vi "Get Paths Array GUI.vi"(9 "Types (string)":string[](array[string]), 10 "Data":string[](array[string])) -> ()   [LabVIEW 2013, in "Data.PGSQL.lvclass"]
uses:
  Data.PGSQL.lvclass
  Typedefs/Errors--enum.ctl
  <userlib>/_OpenG.lib/array/array.llb/Search 1D Array (String)__ogtk.vi
panel:
  out "selected_paths":string
  in  "UNDO LAST VALUE":bool
  out "Paths":string[](array[string])
  out "Message":string
  out "path_to_selected_column":string="llab_038:d001(TEST_TABLE--new_stuff(hippos))"
  out "selected_table":string="TEST_TABLE"
  in  "columns_list":i32(listbox)=1
  in  "tables_list":i32(listbox)=34
  in  "STOP":bool
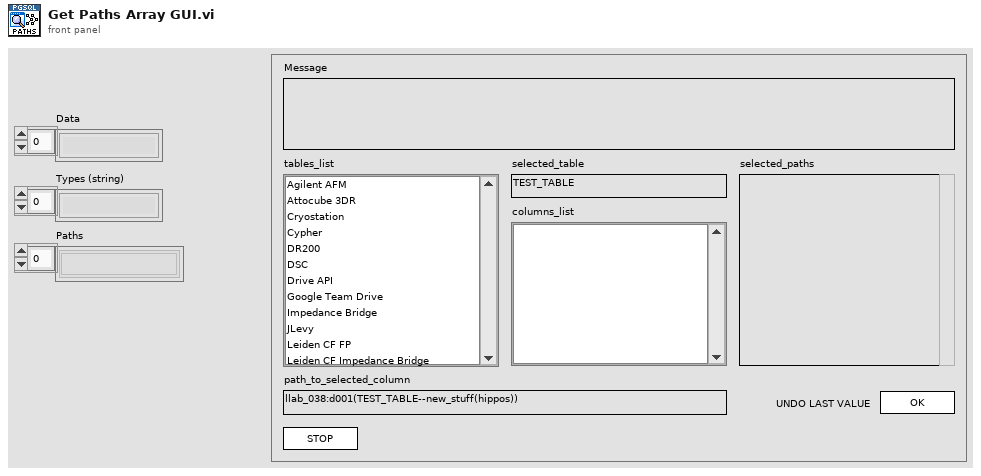
[diagram p1: front panel]
types:
  T1 = enum32{"Invalid", "Standard", "Closed", "Hidden", "Minimized", "Maximized"}
  T2 = enum32{"invalid app kind", "Development System", "Run Time System", "Student Edition", "Embedded LabVIEW", "Evaluation", "Custom"}
  T3 = typedef "Data.PGSQL.lvclass/Errors--enum.ctl" = enum16{"0: None", "5005: Path Type Not Supported", "5006: Number of Variables", "5008: Cannot write two data points", "5030: Start and End Times Identical", "5031: Input is not wholly", "5033: Bad path or paths", "5040: Invalid Instrument Name", "5050: Column can only hold string", "5051 Column can only hold bool", "5052: Column can only hold double", "5053: Column can only hold int"}
  T4 = cluster{"Core":cluster{"Current VI Reference":refnum<vi>, "Close Panel on Exit?":bool}, "Data.PG in":refnum<class "Data.PGSQL.lvclass">, "table names":string[], "table paths":string[], "column names":string[], "column units":string[], "column paths":string[], "new table name":string, "new column name":string, "new column data type":string, "new column units":string, "selected table":string, "selected column":string, "selected table path":string, "selected column path":string, "selected column units":string, "Paths array":string[], "Current Index":i32, "Data":string[], "Types (string)":string[]}
  T5 = cluster{"Current VI Reference":refnum<vi>, "Close Panel on Exit?":bool}
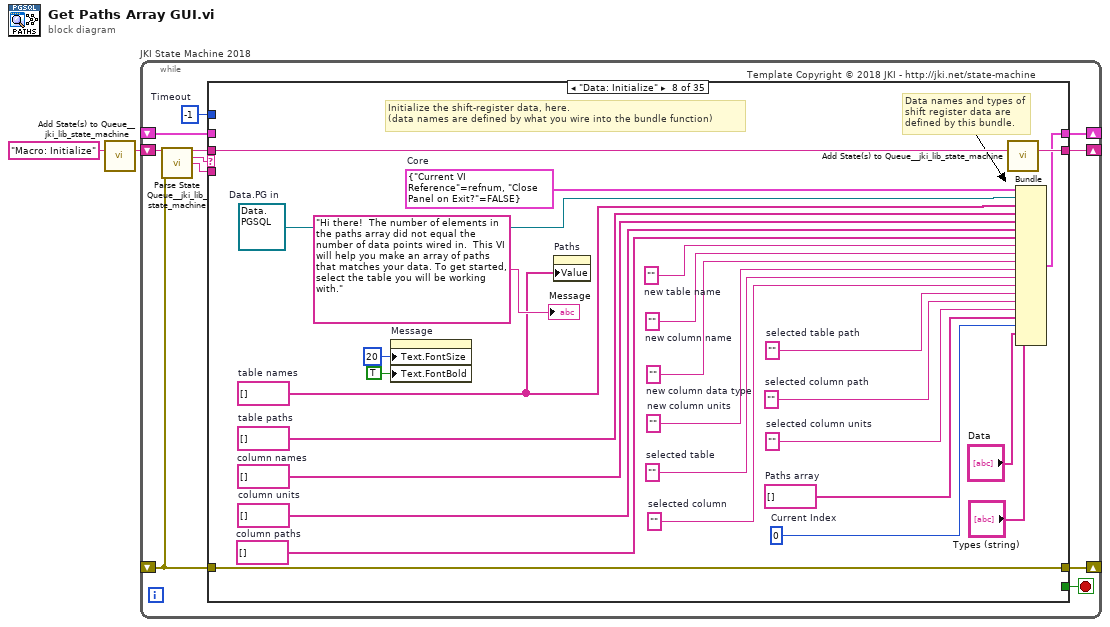
[diagram p0: block diagram]
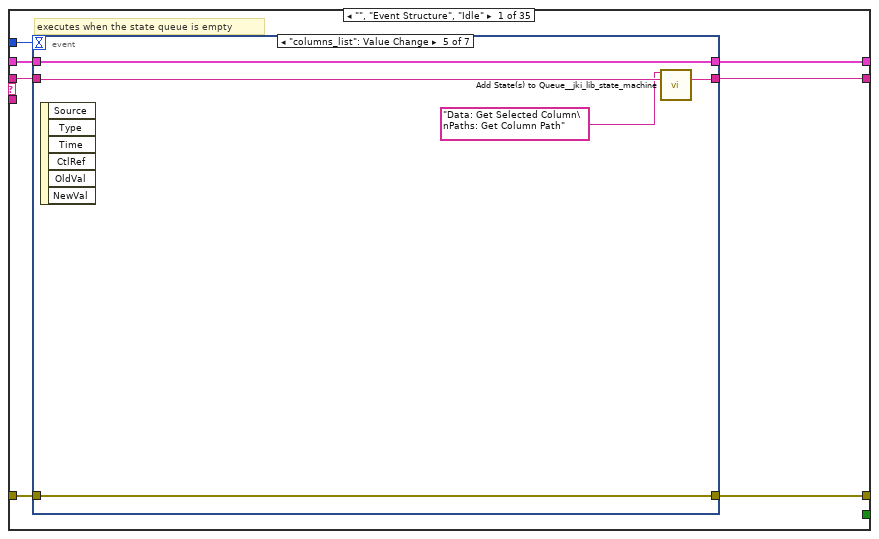
[diagram p2: hidden frame]
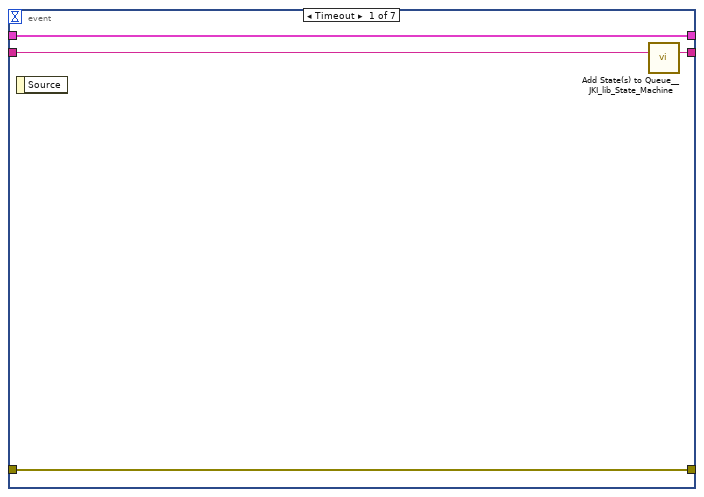
[diagram p3: hidden frame]
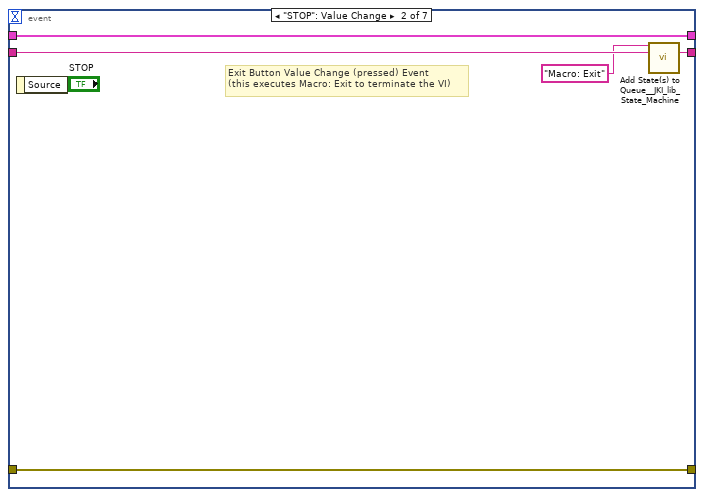
[diagram p4: hidden frame]
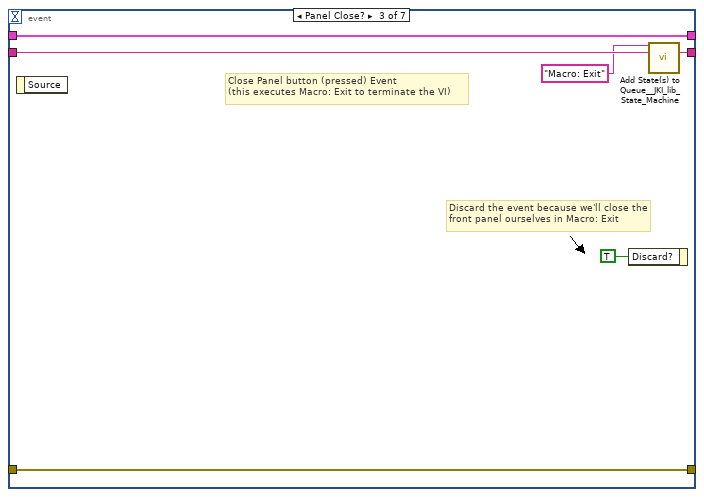
[diagram p5: hidden frame]
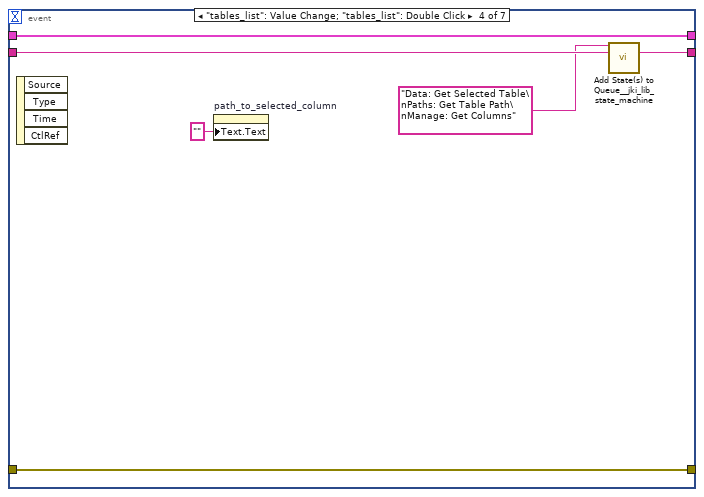
[diagram p6: hidden frame]
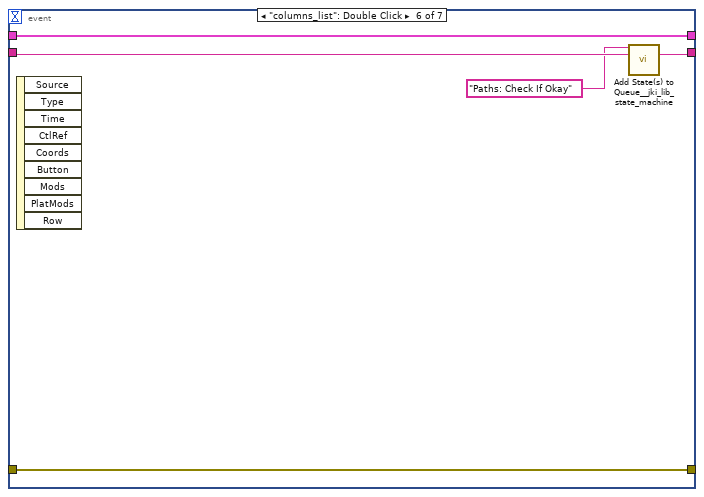
[diagram p7: hidden frame]
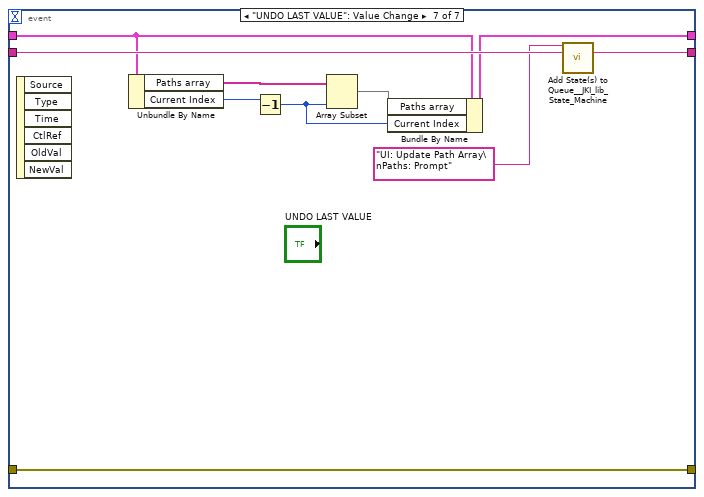
[diagram p8: hidden frame]
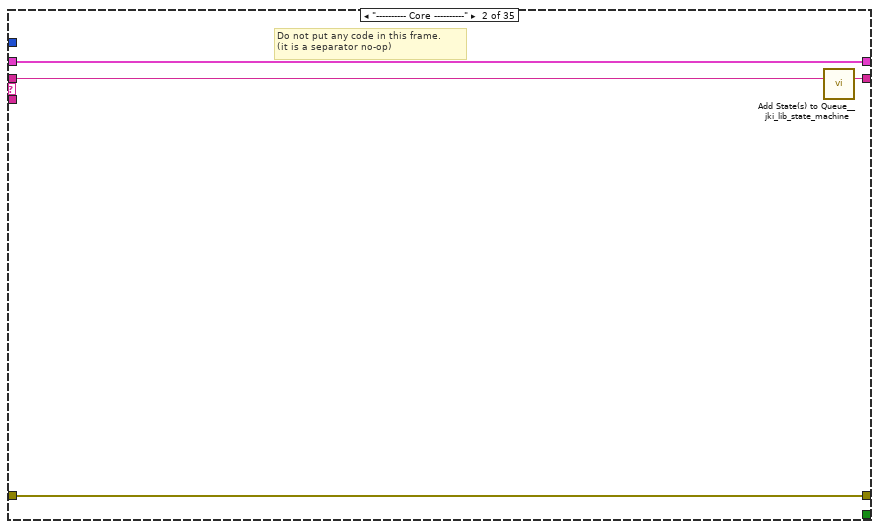
[diagram p9: hidden frame]
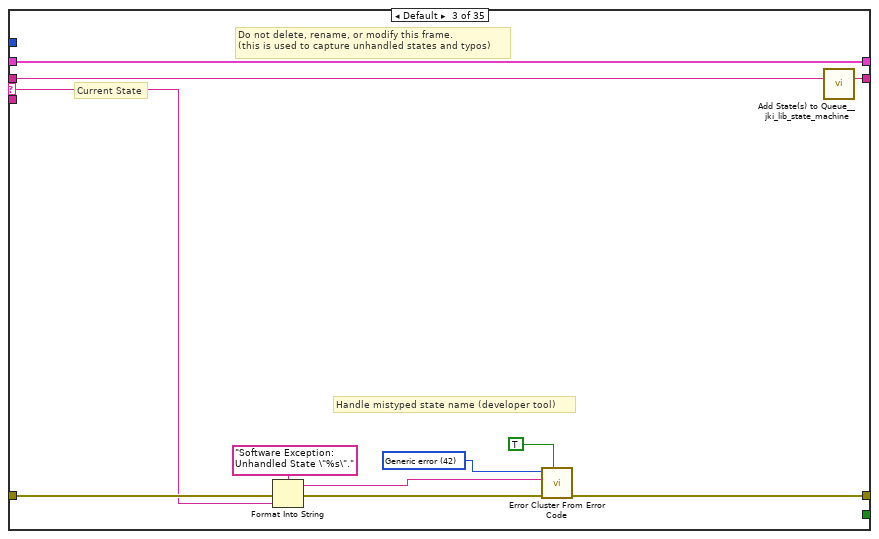
[diagram p10: hidden frame]
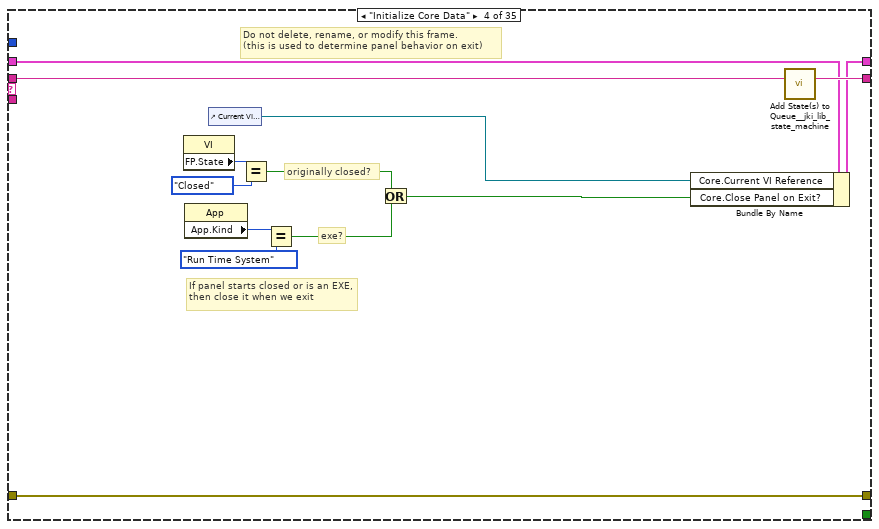
[diagram p11: hidden frame]
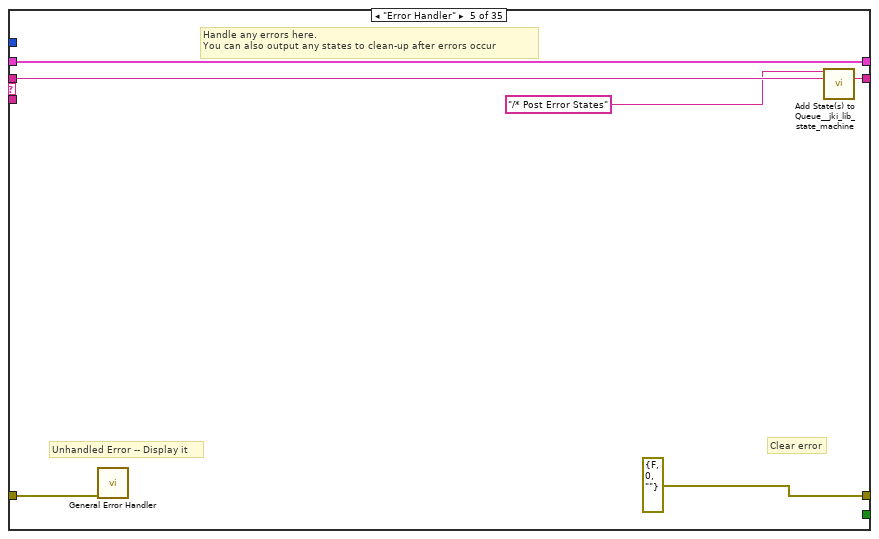
[diagram p12: hidden frame]
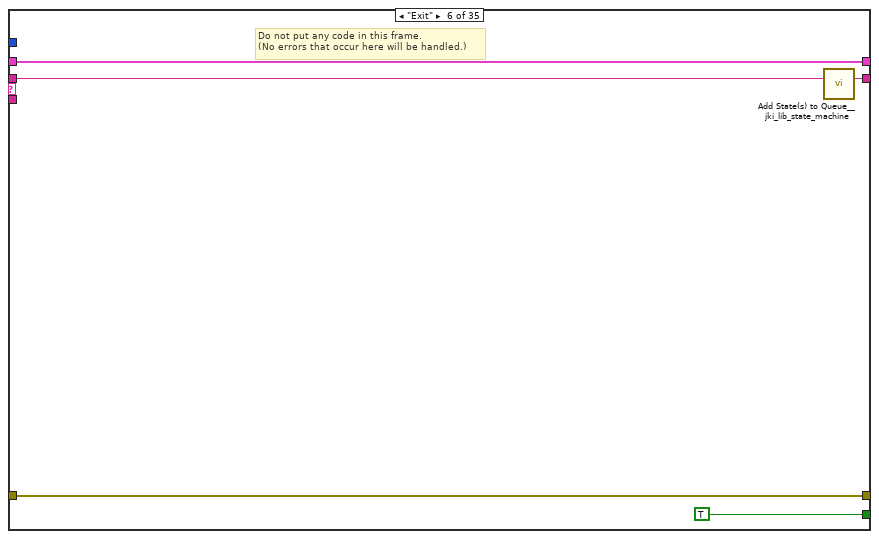
[diagram p13: hidden frame]
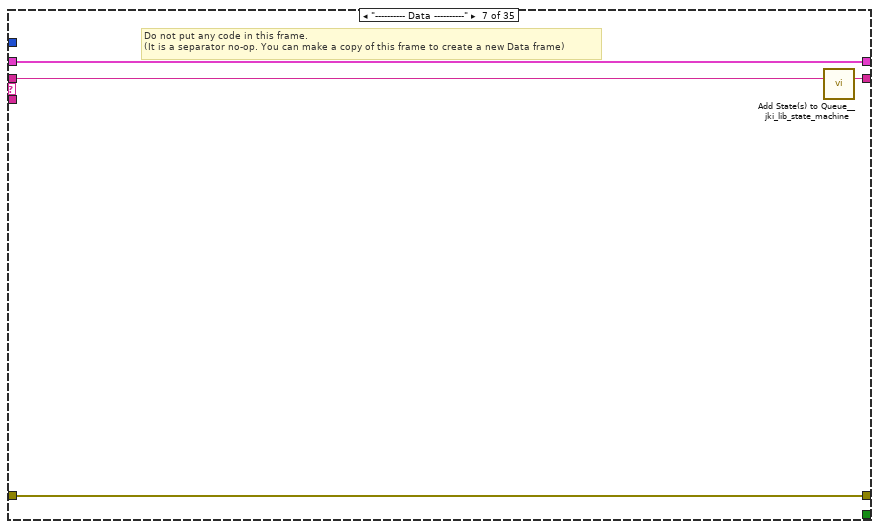
[diagram p14: hidden frame]
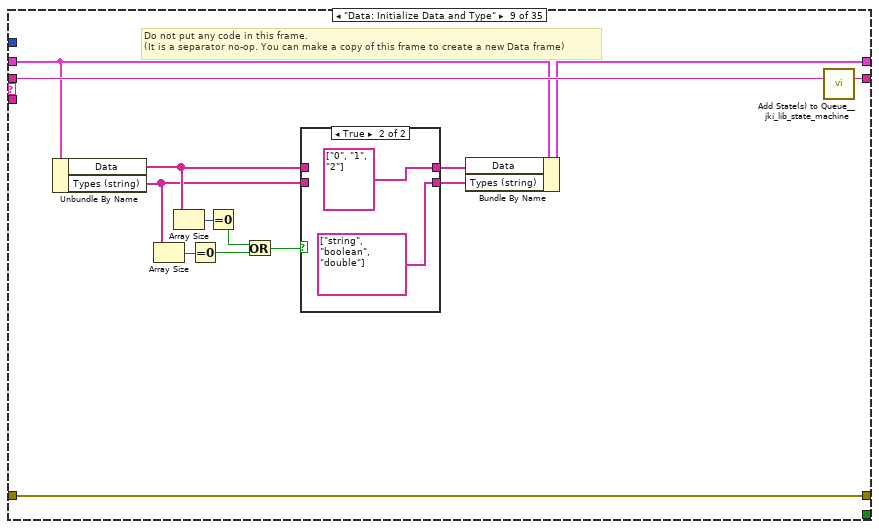
[diagram p15: hidden frame]
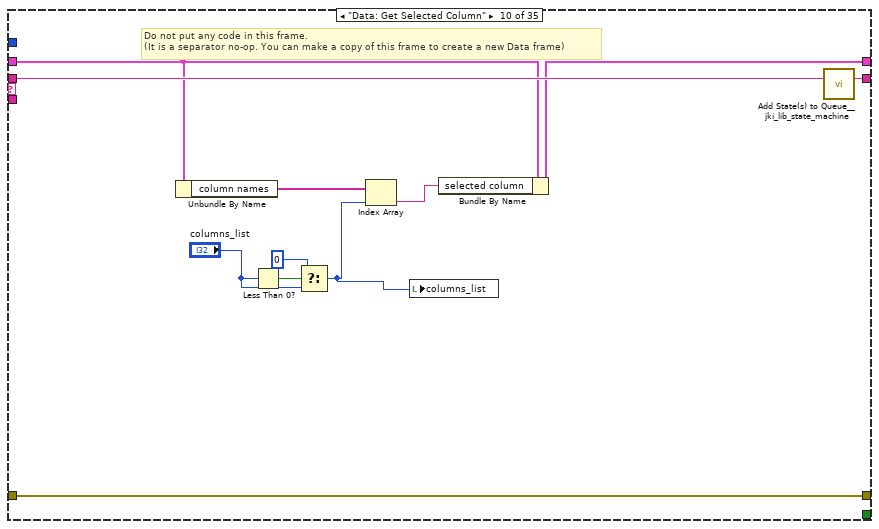
[diagram p17: hidden frame]
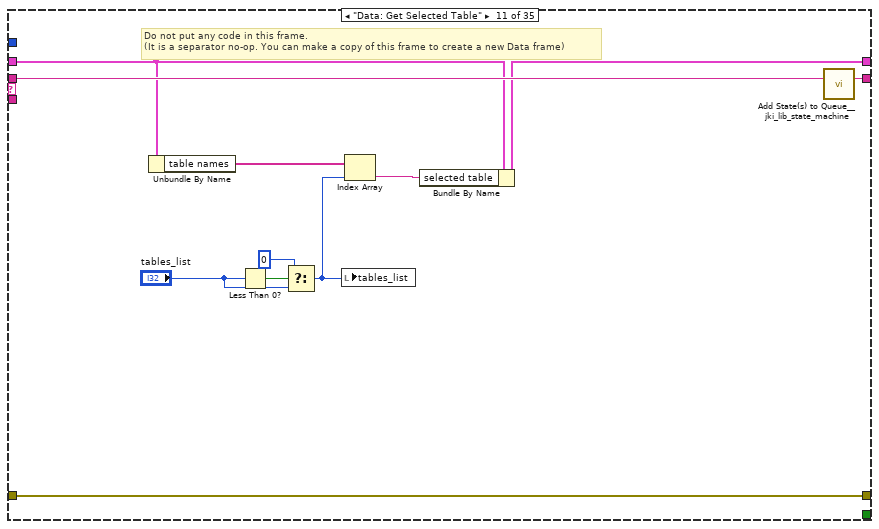
[diagram p18: hidden frame]
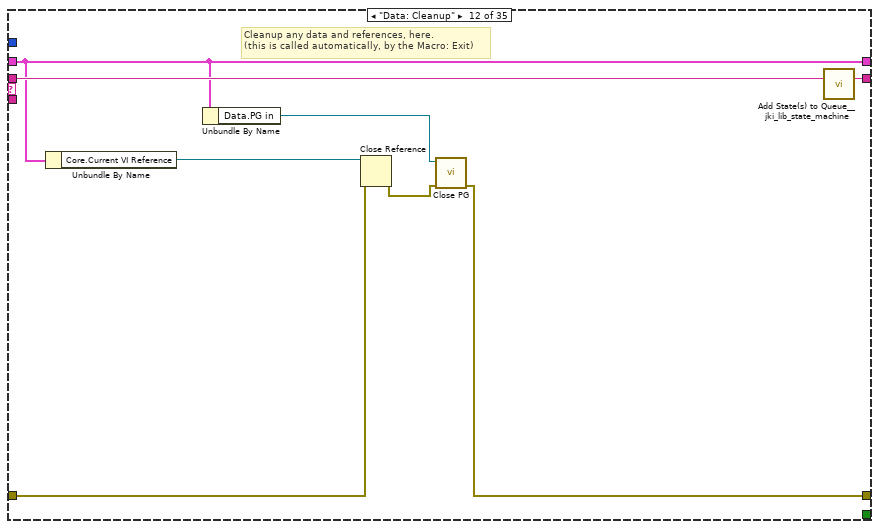
[diagram p19: hidden frame]
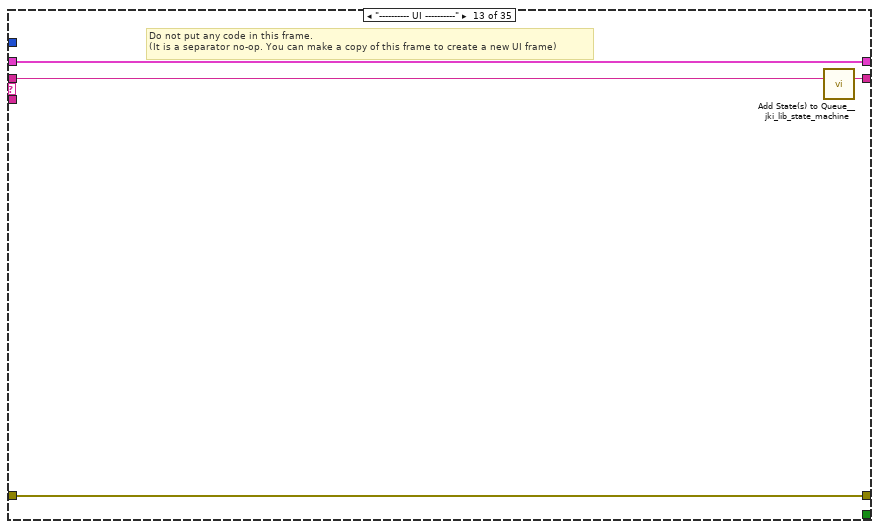
[diagram p20: hidden frame]
diagram:
  n1 = call <vilib>:"Add State(s) to Queue__jki_lib_state_machine.vi"("State(s) in (\"\")"="Macro: Initialize") -> ("States Out"=w2:string)  [unwired: 14 in]
  n2 = while "JKI State Machine 2018" {
    shift-right: [w6] -> _
    shift-left: _ -> [w5]
    shift-right: [w9] -> _
    shift-left: _ -> [w3]
    shift-right: [w8] -> _
    shift-left: w2 -> [w10]
    stop <- w7 stop-if-true
    w4 = -1  # Timeout
    # "Template Copyright © 2018 JKI - http://jki.net/state-machine"
    n3 = call <vilib>:"Parse State Queue__jki_lib_state_machine.vi"("State Queue"=w10, "Error In (no error)"=w3) -> ("Remaining States"=w12:string, "Current State"=w13:string, "Arguments"=w11:string)  [unwired: 11 in]
    n4 = case shown="\"Data: Initialize\"" w13 {
      selector: w13 -> [_ _ w66 _ _ _ _ _ _ _ _ _ _ _ _ _ _ _ _ _ _ _ _ _ _ _ _ _ _ _ _ _ _ _ _]
      tunnel: w12 -> [w20 w65 w70 w89 w95 w100 w104 w131 w145 w160 w171 w179 w183 w194 w202 w208 w219 w291 w296 w305 w309 w314 w324 w328 w337 w350 w354 w360 w368 w372 w381 w395 w406 w425 w461]
      tunnel: w11 -> [_ _ _ _ _ _ _ _ _ _ _ _ _ _ _ w203 w213 _ _ _ _ _ _ _ _ _ _ _ _ _ _ _ _ _ _]
      tunnel: w5 -> [w18 w62 w68 w82 w92 w98 w101 _ w142 w155 w166 w173 w180 w186 w197 w206 w215 w288 w293 w302 w306 w311 w321 w325 w335 w348 w351 w358 w366 w369 w379 w393 w403 w419 w459]
      tunnel: [w17 w63 w72 w86 errorcluster {"status"=FALSE, "code"=0, "source"=""} ("error out") w97 w102 w128 w143 w158 w169 w174 w181 w185 w200 w204 w216 w289 w294 w303 w307 w312 w322 w326 w331 w344 w352 w355 w362 w370 w375 w383 w404 w423 w443] -> w9
      tunnel: w3 -> [w16 w63 w71 w86 w91 w97 w102 w128 w143 w158 w169 w176 w181 w192 w200 w205 w217 w289 w294 w303 w307 w312 w322 w326 w332 w345 w352 w356 w361 w370 w376 w384 w404 w423 w440]
      tunnel: [w19 w64 w69 w88 w94 w99 w103 w130 w144 w159 w170 w178 w182 w193 w201 w207 w218 w290 w295 w304 w308 w313 w323 w327 w336 w349 w353 w359 w367 w371 w380 w394 w405 w424 w460] -> w8
      tunnel: [_ _ _ _ _ TRUE _ _ _ _ _ _ _ _ _ _ _ _ _ _ _ _ _ _ _ _ _ _ _ _ _ _ _ _ _] -> w7
      tunnel: [w15 w62 w68 w87 w92 w98 w101 w129 w141 w156 w165 w173 w180 w186 w197 w206 w215 w288 w293 w302 w306 w311 w321 w325 w334 w347 w351 w358 w365 w369 w373 w385 w403 w408 w459] -> w6
      tunnel: w4 -> [w14 _ _ _ _ _ _ _ _ _ _ _ _ _ _ _ _ _ _ _ _ _ _ _ _ _ _ _ _ _ _ _ _ _ _]
      frame "", "Event Structure", "Idle" {
        # "executes when the state queue is empty"
        n5 = event shown="[4] \"columns_list\": Value Change" {
          selector: _ -> [_ _ _ _ _ _ _]
          dyn-events: _ -> [_ _ _ _ _ _ _]
          timeout: w14 -> [_ _ _ _ _ _ _]
          tunnel: w20 -> [w24 w29 w35 w39 w44 w49 w59]
          tunnel: [w23 w28 w34 w40 w45 w50 w60] -> w19
          tunnel: w18 -> [w21 w26 w32 w36 w46 w48 w56]
          tunnel: [w22 w27 w33 w41 w42 w51 w61] -> w17
          tunnel: w16 -> [w22 w27 w33 w41 w42 w51 w61]
          tunnel: [w21 w26 w32 w36 w46 w48 w55] -> w15
          event Timeout {
            n6 = event-data() -> ()  [unwired: 1 in, 1 out]
            n7 = call <vilib>:"Add State(s) to Queue__JKI_lib_State_Machine.vi"("State(s) in (\"\")"=w24) -> ("States Out"=w23:string)  [unwired: 14 in]
          }
          event "STOP": Value Change {
            # "Exit Button Value Change (pressed) Event\n(this executes Macro: Exit to terminate the VI)"
            n8 = event-data() -> ()  [unwired: 1 in, 1 out]
            n9 = call <vilib>:"Add State(s) to Queue__JKI_lib_State_Machine.vi"("State(s) in Front (\"\")"="Macro: Exit", "State(s) in (\"\")"=w29) -> ("States Out"=w28:string)  [unwired: 13 in]
          }
          event Panel Close? {
            # "Discard the event because we'll close the front panel ourselves in Macro: Exit"
            # "Close Panel button (pressed) Event\n(this executes Macro: Exit to terminate the VI)"
            n10 = event-data() -> ()  [unwired: 1 in, 1 out]
            n11 = event-data("Discard?"=TRUE) -> ()  [unwired: 1 in, 1 out]
            n12 = call <vilib>:"Add State(s) to Queue__JKI_lib_State_Machine.vi"("State(s) in Front (\"\")"="Macro: Exit", "State(s) in (\"\")"=w35) -> ("States Out"=w34:string)  [unwired: 13 in]
          }
          event "tables_list": Value Change; "tables_list": Double Click {
            n13 = event-data() -> ()  [unwired: 1 in, 4 out]
            n14 = property on="path_to_selected_column" class="Str"("Text.Text"="") -> ()  [unwired: 2 in, 2 out]
            n15 = call <vilib>:"Add State(s) to Queue__jki_lib_state_machine.vi"("State(s) in Front (\"\")"="Data: Get Selected Table\nPaths: Get Table Path\nManage: Get Columns" ("State(s) in Front (\"\")"), "State(s) in (\"\")"=w39) -> ("States Out"=w40:string)  [unwired: 13 in]
          }
          event "columns_list": Value Change {
            n16 = event-data() -> ()  [unwired: 1 in, 6 out]
            n17 = call <vilib>:"Add State(s) to Queue__jki_lib_state_machine.vi"("State(s) in Front (\"\")"="Data: Get Selected Column\nPaths: Get Column Path", "State(s) in (\"\")"=w44) -> ("States Out"=w45:string)  [unwired: 13 in]
          }
          event "columns_list": Double Click {
            n18 = event-data() -> ()  [unwired: 1 in, 9 out]
            n19 = call <vilib>:"Add State(s) to Queue__jki_lib_state_machine.vi"("State(s) in Front (\"\")"="Paths: Check If Okay" ("State(s) in Front (\"\")"), "State(s) in (\"\")"=w49) -> ("States Out"=w50:string)  [unwired: 13 in]
          }
          event "UNDO LAST VALUE": Value Change {
            n20 = event-data() -> ()  [unwired: 1 in, 6 out]
            n21 = Unbundle By Name(w56) -> ("Paths array"=w57:string[], "Current Index"=w58:i32)
            n22 = Decrement(x=w58) -> (x-1=w54:i32)
            n23 = Array Subset(array=w57, length=w54) -> (w53:string[])  [unwired: 1 in]
            n24 = Bundle By Name(cluster=w56, "Paths array"=w53, "Current Index"=w54) -> (w55:T4)
            n25 = call <vilib>:"Add State(s) to Queue__JKI_lib_State_Machine.vi"("State(s) in Front (\"\")"="UI: Update Path Array\nPaths: Prompt" ("State(s) in Front (\"\")"), "State(s) in (\"\")"=w59) -> ("States Out"=w60:string)  [unwired: 13 in]
          }
        }
      }
      frame "---------- Core ----------" {
        # "Do not put any code in this frame.\n(it is a separator no-op)"
        n26 = call <vilib>:"Add State(s) to Queue__jki_lib_state_machine.vi"("State(s) in (\"\")"=w65) -> ("States Out"=w64:string)  [unwired: 14 in]
      }
      frame Default {
        w75 = 42 items=["No error", "Argument error", "Memory is full", "Out of zone", "End of file", "File already open", "Generic file I/O error", "File not found", "File permission error", "Disk is full", "Duplicate path", "Too many files open", "System feature not enabled", "Resource file not found", "Cannot add resource", "Resource not found", "Image not found", "Image memory error", "Pen does not exist", "Config type invalid", "Config token not found", "Config parse error", "Config memory error", "Bad external code format", "Bad external code offset", "External code not present", "Null window", "Destroy window error", "Null menu", "Print aborted", "Bad print record", "Print driver error", "Windows error during printing", "Memory error during printing", "Print dialog error", "Generic print error", "Invalid device refnum", "Device not found", "Device parameter error", "Device unit error", "Cannot open device", "Device call aborted", "Generic error", "Cancelled by user", "Object ID too low", "Object ID too high", "Object not in heap", "Unknown heap", "Unknown object (invalid DefProc)", "Unknown object (DefProc not in table)", "Message out of range", "Invalid (null) method", "Unknown message", "Manager call not supported", "Bad address", "Network operation in progress", "Network operation timed out", "Connection is busy", "Network attribute not supported", "Network error", "Address in use", "System out of memory", "Connection aborted", "Connection refused", "Not connected", "Already connected", "Connection closed", "Initialization error (interapplication manager)", "Bad occurrence", "Wait on unbound occurrence handler", "Occurrence queue overflow", "Datalog type conflict", "Unused", "Unrecognized type (interapplication manager)", "Memory corrupt", "Failed to make temporary DLL", "Old CIN version", "Drag socket not found", "Failed to load drop-object", "Failed to register OLE object", "Failed to release OLE object", "Format specifier type mismatch", "Unknown format specifier", "Too few format specifiers", "Too many format specifiers", "Scan failed", "Newer CIN version", "Error converting to variant", "Runtime menu error", "Password tampered", "Variant attribute not found", "Incompatible variant data type", "Event data is not available", "Event Store is not present", "Occurrence is not found", "Event Queue is not created", "Event info is not available", "Refnum passed is NULL", "Error retrieving Class GUID", "Error retrieving CoClass GUID", "Error retrieving TypeLib GUID.", "Bad built application magic bytes.", "Specific driver is different from the specific driver associated with the Logical Name.", "There is no session opened to the class driver.", "Max Error", "MAX - Error with config objects", "MAX - Error loading configuration", "MAX - Group not supported"]
        # "Current State"
        # "Do not delete, rename, or modify this frame.\n(this is used to capture unhandled states and typos)"
        # "Handle mistyped state name (developer tool)"
        n27 = Format Into String(format string="Software Exception: Unhandled State \"%s\"." ("message"), error in=w71, w66) -> (resulting string=w74:string, error out=w73:errorcluster)  [unwired: 1 in]
        n28 = call <vilib>:"Error Cluster From Error Code.vi"("show call chain? (False)"=TRUE, "error in (no error)"=w73, "error message (\"\")"=w74, "error code (0)"=w75) -> ("error out"=w72:errorcluster)  [unwired: 5 in]
        n29 = call <vilib>:"Add State(s) to Queue__jki_lib_state_machine.vi"("State(s) in (\"\")"=w70) -> ("States Out"=w69:string)  [unwired: 14 in]
      }
      frame "Initialize Core Data" {
        # "Do not delete, rename, or modify this frame.\n(this is used to determine panel behavior on exit)"
        # "originally closed?"
        # "exe?"
        # "If panel starts closed or is an EXE, then close it when we exit"
        n30 = property class="VI"() -> ("FP.State"=w79:T1)  [unwired: 2 in, 2 out]
        n31 = property class="App"() -> ("App.Kind"=w85:T2)  [unwired: 2 in, 2 out]
        n32 = control-ref of="Current VI Reference"() -> (w80:refnum<vi>)
        n33 = Equal?(x=w79, y=T1."Closed" ("Front Panel Window:State")) -> (x = y?=w77:bool)
        n34 = Equal?(x=w85, y=T2."Run Time System" ("Application:Kind")) -> (x = y?=w83:bool)
        n35 = Or(x=w77, y=w83) -> (x .or. y?=w81:bool)
        n36 = Bundle By Name(cluster=w82, "Core.Current VI Reference"=w80, "Core.Close Panel on Exit?"=w81) -> (w87:T4)
        n37 = call <vilib>:"Add State(s) to Queue__jki_lib_state_machine.vi"("State(s) in (\"\")"=w89) -> ("States Out"=w88:string)  [unwired: 14 in]
      }
      frame "Error Handler" {
        # "Unhandled Error -- Display it"
        # "Handle any errors here.\nYou can also output any states to clean-up after errors occur"
        # "Clear error"
        n38 = call <vilib>:"General Error Handler.vi"("error in (no error)"=w91) -> ()  [unwired: 10 in, 5 out]
        n39 = call <vilib>:"Add State(s) to Queue__jki_lib_state_machine.vi"("State(s) in Front (\"\")"="/* Post Error States", "State(s) in (\"\")"=w95) -> ("States Out"=w94:string)  [unwired: 13 in]
      }
      frame "Exit" {
        # "Do not put any code in this frame.\n(No errors that occur here will be handled.)"
        n40 = call <vilib>:"Add State(s) to Queue__jki_lib_state_machine.vi"("State(s) in (\"\")"=w100) -> ("States Out"=w99:string)  [unwired: 14 in]
      }
      frame "---------- Data ----------" {
        # "Do not put any code in this frame.\n(It is a separator no-op. You can make a copy of this frame to create a new Data frame)"
        n41 = call <vilib>:"Add State(s) to Queue__jki_lib_state_machine.vi"("State(s) in (\"\")"=w104) -> ("States Out"=w103:string)  [unwired: 14 in]
      }
      frame "Data: Initialize" {
        w112 = 0  # Current Index
        w113 = string[] []  # Paths array
        w114 = ""  # selected column units
        w105 = ""  # selected column path
        w115 = ""  # selected table path
        w116 = ""  # selected column
        w117 = ""  # selected table
        w118 = ""  # new column units
        w119 = ""  # new column data type
        w120 = ""  # new column name
        w121 = ""  # new table name
        w122 = string[] []  # column paths
        w123 = string[] []  # column units
        w124 = string[] []  # column names
        w125 = string[] []  # table paths
        w106 = string[] []  # table names
        w126 = refnum<class "Data.PGSQL.lvclass"> refnum  # Data.PG in
        w127 = T5 {"Current VI Reference"=refnum, "Close Panel on Exit?"=FALSE}  # Core
        # "Data names and types of shift register data are defined by this bundle."
        # "Initialize the shift-register data, here.\n(data names are defined by what you wire into the bundle function)"
        n42 = property on="Message" class="Str"("Text.FontSize"=u32 20 ("Text.Font:Size"), "Text.FontBold"=TRUE ("Text.Font:Bold")) -> ()  [unwired: 2 in, 2 out]
        n43 = property on="Paths" class="Arr (strict)"("Value"=w106) -> ()  [unwired: 2 in, 2 out]
        n44 = call <vilib>:"Add State(s) to Queue__jki_lib_state_machine.vi"("State(s) in (\"\")"=w131) -> ("States Out"=w130:string)  [unwired: 14 in]
        n45 = Bundle("Core"=w127, "Data.PG in"=w126, "table names"=w106, "table paths"=w125, "column names"=w124, "column units"=w123, "column paths"=w122, "new table name"=w121, "new column name"=w120, "new column data type"=w119, "new column units"=w118, "selected table"=w117, "selected column"=w116, "selected table path"=w115, "selected column path"=w105, "selected column units"=w114, "Paths array"=w113, "Current Index"=w112, "Data"="Data", "Types (string)"="Types (string)") -> (w129:T4)  [unwired: 1 in]
        "Message" <- "Hi there!  The number of elements in the paths array did not equal the number of data points wired in.  This VI will help you make an array of paths that matches your data. To get started, select the table you will be working with." ("String")
      }
      frame "Data: Initialize Data and Type" {
        # "Do not put any code in this frame.\n(It is a separator no-op. You can make a copy of this frame to create a new Data frame)"
        n46 = Unbundle By Name(w142) -> ("Data"=w134:string[], "Types (string)"=w132:string[])
        n47 = Array Size(array=w132) -> (size(s)=w139:i32)
        n48 = Array Size(array=w134) -> (size(s)=w140:i32)
        n49 = Equal To 0?(x=w139) -> (x = 0?=w137:bool)
        n50 = Equal To 0?(x=w140) -> (x = 0?=w138:bool)
        n51 = Or(x=w138, y=w137) -> (x .or. y?=w136:bool)
        n52 = case shown="True" w136 {
          tunnel: [w147 string[] ["0", "1", "2"] ("Data")] -> w135
          tunnel: w134 -> [w147 _]
          tunnel: [w146 string[] ["string", "boolean", "double"] ("Types (string)")] -> w133
          tunnel: w132 -> [w146 _]
          frame False {
          }
          frame True {
          }
        }
        n53 = Bundle By Name(cluster=w142, "Data"=w135, "Types (string)"=w133) -> (w141:T4)
        n54 = call <vilib>:"Add State(s) to Queue__jki_lib_state_machine.vi"("State(s) in (\"\")"=w145) -> ("States Out"=w144:string)  [unwired: 14 in]
      }
      frame "Data: Get Selected Column" {
        # "Do not put any code in this frame.\n(It is a separator no-op. You can make a copy of this frame to create a new Data frame)"
        n55 = Unbundle By Name(w155) -> ("column names"=w157:string[])
        n56 = Less Than 0?(x="columns_list") -> (x < 0?=w153:bool)
        n57 = Select(t=0, s=w153, f="columns_list") -> (s? t:f=w150:i32)
        n58 = Index Array(array=w157, index=w150) -> (element=w151:string)
        n59 = local write "columns_list"(w150) -> ()
        n60 = Bundle By Name(cluster=w155, "selected column"=w151) -> (w156:T4)
        n61 = call <vilib>:"Add State(s) to Queue__jki_lib_state_machine.vi"("State(s) in (\"\")"=w160) -> ("States Out"=w159:string)  [unwired: 14 in]
      }
      frame "Data: Get Selected Table" {
        # "Do not put any code in this frame.\n(It is a separator no-op. You can make a copy of this frame to create a new Data frame)"
        n62 = Unbundle By Name(w166) -> ("table names"=w167:string[])
        n63 = Less Than 0?(x="tables_list") -> (x < 0?=w163:bool)
        n64 = Select(t=0, s=w163, f="tables_list") -> (s? t:f=w161:i32)
        n65 = local write "tables_list"(w161) -> ()
        n66 = Index Array(array=w167, index=w161) -> (element=w168:string)
        n67 = Bundle By Name(cluster=w166, "selected table"=w168) -> (w165:T4)
        n68 = call <vilib>:"Add State(s) to Queue__jki_lib_state_machine.vi"("State(s) in (\"\")"=w171) -> ("States Out"=w170:string)  [unwired: 14 in]
      }
      frame "Data: Cleanup" {
        # "Cleanup any data and references, here.\n(this is called automatically, by the Macro: Exit)"
        n69 = Unbundle By Name(w173) -> ("Core.Current VI Reference"=w177:refnum<vi>)
        n70 = Unbundle By Name(w173) -> ("Data.PG in"=w172:refnum<class "Data.PGSQL.lvclass">)
        n71 = Close Reference(reference=w177, error in (no error)=w176) -> (error out=w175:errorcluster)
        n72 = call-dynamic "Close PG.vi"("error in (no error)"=w175, "Data.PG in"=w172) -> ("error out"=w174:errorcluster)  [unwired: 8 in, 1 out]
        n73 = call <vilib>:"Add State(s) to Queue__jki_lib_state_machine.vi"("State(s) in (\"\")"=w179) -> ("States Out"=w178:string)  [unwired: 14 in]
      }
      frame "---------- UI ----------" {
        # "Do not put any code in this frame.\n(It is a separator no-op. You can make a copy of this frame to create a new UI frame)"
        n74 = call <vilib>:"Add State(s) to Queue__jki_lib_state_machine.vi"("State(s) in (\"\")"=w183) -> ("States Out"=w182:string)  [unwired: 14 in]
      }
      frame "UI: Initialize" {
        w184 = "" ("Text.Text")
        # "Initialize the User Interface, here.\n(this is called automatically, by the Macro: Init)"
        n75 = Unbundle By Name(w186) -> ("table names"=w191:string[], "column names"=w190:string[], "selected table"=→"selected_table":string)
        n76 = call <userlib>:"Fit VI window to Largest Dec__ogtk.vi"("error in (no error)"=w192) -> ("error out"=w185:errorcluster)  [unwired: 5 in, 1 out]
        n77 = property on="tables_list" class="LstBox (strict)"("Item Names"=w191) -> ()  [unwired: 2 in, 2 out]
        n78 = Build Array(0) -> (w187:i32[])
        n79 = property on="path_to_selected_column" class="Str"("Text.Text"=w184) -> ()  [unwired: 2 in, 2 out]
        n80 = local write "selected_paths"(w184) -> ()
        n81 = property on="Paths" class="Arr (strict)"("Index Values"=w187) -> ()  [unwired: 2 in, 2 out]
        n82 = property on="columns_list" class="LstBox (strict)"("Item Names"=w190) -> ()  [unwired: 2 in, 2 out]
        n83 = call <vilib>:"Add State(s) to Queue__jki_lib_state_machine.vi"("State(s) in (\"\")"=w194) -> ("States Out"=w193:string)  [unwired: 14 in]
      }
      frame "UI: Update" {
        # "Initialize the User Interface, here.\n(this is called automatically, by the Macro: Init)"
        n84 = Unbundle By Name(w197) -> ("table names"=w199:string[], "column names"=w198:string[], "selected table"=w195:string, "selected column"=w196:string)
        n85 = local write "selected_table"(w195) -> ()
        n86 = property on="tables_list" class="LstBox (strict)"("Item Names"=w199) -> ()  [unwired: 2 in, 2 out]
        n87 = property on="path_to_selected_column" class="Str"("Text.Text"=w196) -> ()  [unwired: 2 in, 2 out]
        n88 = property on="columns_list" class="LstBox (strict)"("Item Names"=w198) -> ()  [unwired: 2 in, 2 out]
        n89 = call <vilib>:"Add State(s) to Queue__jki_lib_state_machine.vi"("State(s) in (\"\")"=w202) -> ("States Out"=w201:string)  [unwired: 14 in]
      }
      frame "UI: Cursor Set" {
        # "Argument"
        # "Set and Unset Cursor Busy.\n(Usage: \"UI: Cursor Set >> Busy|Idle\")"
        n90 = case shown="\"Idle\", Default" w203 {
          tunnel: w205 -> [w210 w212]
          tunnel: [w209 w211] -> w204
          frame "Idle", Default {
            n91 = call <vilib>:"Unset Busy.vi"("error in (no error)"=w210) -> ("error out"=w209:errorcluster)  [unwired: 10 in]
          }
          frame "Busy" {
            n92 = call <vilib>:"Set Busy.vi"("error in (no error)"=w212) -> ("error out"=w211:errorcluster)  [unwired: 9 in, 1 out]
          }
        }
        n93 = call <vilib>:"Add State(s) to Queue__jki_lib_state_machine.vi"("State(s) in (\"\")"=w208) -> ("States Out"=w207:string)  [unwired: 14 in]
      }
      frame "UI: Front Panel State" {
        # "Argument"
        # "Set Front Panel Open or Closed\n(Usage: \"UI: Front Panel State >> Open|Close\")"
        n94 = Unbundle By Name(w215) -> ("Core.Current VI Reference"=w214:refnum<vi>)
        n95 = case shown="\"Maximize\", \"Maximized\"" w213 {
          tunnel: w217 -> [w225 w240 w251 w264 w277]
          tunnel: [w227 w241 w253 w266 w279] -> w216
          tunnel: w214 -> [w226 w238 w252 w265 w278]
          frame "Open", "Standard", Default {
            w220 = T1."Standard" ("State")
            n96 = property class="VI"(reference=w226, error in=w225) -> (reference out=w223:refnum<vi>, error out=w224:errorcluster, "FP.State"=w222:T1)
            n97 = Not Equal?(x=w222, y=w220) -> (x != y?=w221:bool)
            n98 = case shown="True" w221 {
              tunnel: [w231 w233] -> w227
              tunnel: w224 -> [w230 w233]
              tunnel: w223 -> [w229 _]
              tunnel: w220 -> [w228 _]
              frame True {
                n99 = invoke class="VI" method="FP.Open"(reference=w229, error in=w230, "Activate"=TRUE, "State"=w228) -> (error out=w231:errorcluster)  [unwired: 1 in, 4 out]
              }
              frame False {
              }
            }
          }
          frame "Close", "Closed" {
            n100 = property class="VI"(reference=w238, error in=w240) -> (reference out=w237:refnum<vi>, error out=w239:errorcluster, "FP.State"=w235:T1)
            n101 = Not Equal?(x=w235, y=T1."Closed" ("Front Panel Window:State")) -> (x != y?=w234:bool)
            n102 = case shown="True" w234 {
              tunnel: [w242 w245] -> w241
              tunnel: w239 -> [w242 w244]
              tunnel: w237 -> [_ w243]
              frame False {
              }
              frame True {
                n103 = invoke class="VI" method="FP.Close"(reference=w243, error in=w244) -> (error out=w245:errorcluster)  [unwired: 1 in, 2 out]
              }
            }
          }
          frame "Hidden", "Hide" {
            w246 = T1."Hidden" ("State")
            n104 = property class="VI"(reference=w252, error in=w251) -> (reference out=w249:refnum<vi>, error out=w250:errorcluster, "FP.State"=w248:T1)
            n105 = Not Equal?(x=w248, y=w246) -> (x != y?=w247:bool)
            n106 = case shown="True" w247 {
              tunnel: [w257 w258] -> w253
              tunnel: w250 -> [w256 w258]
              tunnel: w249 -> [w255 _]
              tunnel: w246 -> [w254 _]
              frame True {
                n107 = invoke class="VI" method="FP.Open"(reference=w255, error in=w256, "State"=w254) -> (error out=w257:errorcluster)  [unwired: 2 in, 4 out]
              }
              frame False {
              }
            }
          }
          frame "Minimize", "Minimized" {
            w259 = T1."Minimized" ("State")
            n108 = property class="VI"(reference=w265, error in=w264) -> (reference out=w262:refnum<vi>, error out=w263:errorcluster, "FP.State"=w261:T1)
            n109 = Not Equal?(x=w261, y=w259) -> (x != y?=w260:bool)
            n110 = case shown="True" w260 {
              tunnel: [w270 w271] -> w266
              tunnel: w263 -> [w269 w271]
              tunnel: w262 -> [w268 _]
              tunnel: w259 -> [w267 _]
              frame True {
                n111 = invoke class="VI" method="FP.Open"(reference=w268, error in=w269, "State"=w267) -> (error out=w270:errorcluster)  [unwired: 2 in, 4 out]
              }
              frame False {
              }
            }
          }
          frame "Maximize", "Maximized" {
            w272 = T1."Maximized" ("State")
            n112 = property class="VI"(reference=w278, error in=w277) -> (reference out=w275:refnum<vi>, error out=w276:errorcluster, "FP.State"=w274:T1)
            n113 = Not Equal?(x=w274, y=w272) -> (x != y?=w273:bool)
            n114 = case shown="True" w273 {
              tunnel: [w283 w284] -> w279
              tunnel: w276 -> [w282 w284]
              tunnel: w275 -> [w281 _]
              tunnel: w272 -> [w280 _]
              frame True {
                n115 = invoke class="VI" method="FP.Open"(reference=w281, error in=w282, "State"=w280) -> (error out=w283:errorcluster)  [unwired: 2 in, 4 out]
              }
              frame False {
              }
            }
          }
        }
        n116 = call <vilib>:"Add State(s) to Queue__jki_lib_state_machine.vi"("State(s) in (\"\")"=w219) -> ("States Out"=w218:string)  [unwired: 14 in]
      }
      frame "UI: Update Path Array" {
        # "Do not put any code in this frame.\n(It is a separator no-op. You can make a copy of this frame to create a new UI frame)"
        n117 = Unbundle By Name(w288) -> ("Paths array"=w286:string[])
        "Paths" <- w286
        n118 = call "1D Array to String__ogtk.vi"("delimiter (Tab)"="\n", "Array of Strings"=w286) -> ("delimited string"=→"selected_paths":string)  [unwired: 9 in]
        n119 = call <vilib>:"Add State(s) to Queue__jki_lib_state_machine.vi"("State(s) in (\"\")"=w291) -> ("States Out"=w290:string)  [unwired: 14 in]
      }
      frame "UI: Wait" {
        # "Do not put any code in this frame.\n(It is a separator no-op. You can make a copy of this frame to create a new UI frame)"
        n120 = Wait (ms)(milliseconds to wait=u32 15000) -> ()  [unwired: 1 out]
        n121 = call <vilib>:"Add State(s) to Queue__jki_lib_state_machine.vi"("State(s) in (\"\")"=w296) -> ("States Out"=w295:string)  [unwired: 14 in]
      }
      frame "UI: Finish" {
        # "Do not put any code in this frame.\n(It is a separator no-op. You can make a copy of this frame to create a new UI frame)"
        n122 = Unbundle By Name(w302) -> ("Paths array"=w301:string[])
        n123 = call "1D Array to String__ogtk.vi"("delimiter (Tab)"="\n", "Array of Strings"=w301) -> ("delimited string"=w300:string)  [unwired: 9 in]
        n124 = property on="Message" class="Str"("Text.Text"="Great work! Your paths have been copied to your clipboard.  Find where you placed Insert.vi, wire a string constant to the control for paths, and paste the text from your clipboard into the string constant.  This VI will close after 15 seconds ") -> ()  [unwired: 2 in, 2 out]
        n125 = invoke class="App" method="Clipboard.Write"("Param 0"=w300) -> ()  [unwired: 3 in, 4 out]
        n126 = call <vilib>:"Add State(s) to Queue__jki_lib_state_machine.vi"("State(s) in Front (\"\")"="UI: Wait" ("State(s) in Front (\"\")"), "State(s) in (\"\")"=w305) -> ("States Out"=w304:string)  [unwired: 13 in]
      }
      frame "---------- Macro ----------" {
        # "Do not put any code in this frame.\n(It is a separator no-op. You can make a copy of this frame to create a new Macro frame)"
        n127 = call <vilib>:"Add State(s) to Queue__jki_lib_state_machine.vi"("State(s) in (\"\")"=w309) -> ("States Out"=w308:string)  [unwired: 14 in]
      }
      frame "Macro: Initialize" {
        w310 = "Data: Initialize\nInitialize Core Data\nUI: Initialize\nUI: Front Panel State >> Open\nData: Initialize Data and Type\n\nConnection: Open\nManage: Get Tables\nUI: Update\n\n//Data: Get Selected Table\n//Paths: Get Table Path\n\n//Manage: Get Columns\n//UI: Update\n//Data: Get Selected Column\n\n//Paths: Get Column Path"  # Data: Initialize Initialize Core Data UI: Initialize UI: Front Panel State >> Open Data: Initialize Data and Type  Connection: Open Manage: Get Tables UI: Update  //Data: Get Selected Table //Paths: Get Table Path  //Manage: Get Columns //UI: Update //Data: Get Selected Column  //Paths: Get Column Path
        # "Initialization Macro\n(This is called once, when the VI starts)"
        n128 = call <vilib>:"Add State(s) to Queue__jki_lib_state_machine.vi"("State(s) in Front (\"\")"=w310, "State(s) in (\"\")"=w314) -> ("States Out"=w313:string)  [unwired: 13 in]
      }
      frame "Macro: Exit" {
        # "Exit Macro\n(This is called once, when the VI exits)"
        n129 = Unbundle By Name(w321) -> ("Core.Close Panel on Exit?"=w320:bool)
        n130 = Select(t="UI: Front Panel State >> Close", s=w320, f="") -> (s? t:f=w317:string)
        n131 = call <vilib>:"Add State(s) to Queue__jki_lib_state_machine.vi"("State(s) in (\"\")"=w317, "State(s) at Back (\"\")"="Data: Cleanup\nConnection: Close\nExit") -> ("States Out"=w315:string)  [unwired: 13 in]
        n132 = call <vilib>:"Add State(s) to Queue__jki_lib_state_machine.vi"("State(s) in Front (\"\")"=w315, "State(s) in (\"\")"=w324) -> ("States Out"=w323:string)  [unwired: 13 in]
      }
      frame "---------- Manage ----------" {
        # "Template Separator\n(You can make a copy of, or modify, this frame)"
        n133 = call <vilib>:"Add State(s) to Queue__jki_lib_state_machine.vi"("State(s) in (\"\")"=w328) -> ("States Out"=w327:string)  [unwired: 14 in]
      }
      frame "Manage: Get Tables" {
        # "Your code here.\n(You can make a copy of, or modify, this frame)"
        n134 = Unbundle By Name(w335) -> ("Data.PG in"=w333:refnum<class "Data.PGSQL.lvclass">)
        n135 = call "Get Tables.vi"("error in (no error)"=w332, "Data.PG"=w333) -> ("error out"=w331:errorcluster, "Table Paths"=w329:string[], "Table Names"=w330:string[])  [unwired: 6 in, 1 out]
        n136 = Bundle By Name(cluster=w335, "table names"=w330, "table paths"=w329) -> (w334:T4)
        n137 = call <vilib>:"Add State(s) to Queue__jki_lib_state_machine.vi"("State(s) in (\"\")"=w337) -> ("States Out"=w336:string)  [unwired: 14 in]
      }
      frame "Manage: Get Columns" {
        # "Your code here.\n(You can make a copy of, or modify, this frame)"
        n138 = Unbundle By Name(w348) -> ("Data.PG in"=w343:refnum<class "Data.PGSQL.lvclass">, "selected table path"=w342:string)
        n139 = call "Get Columns.vi"("error in (no error)"=w345, "selected table path"=w342, "Data.PG in"=w343) -> ("error out"=w344:errorcluster, "Column Paths"=w339:string[], "Column Names"=w341:string[], "Data.PG out"=w340:refnum<class "Data.PGSQL.lvclass">, "Column Units"=w338:string[])  [unwired: 4 in]
        n140 = Bundle By Name(cluster=w348, "Data.PG in"=w340, "column names"=w341, "column paths"=w339, "column units"=w338) -> (w347:T4)
        n141 = call <vilib>:"Add State(s) to Queue__jki_lib_state_machine.vi"("State(s) in Front (\"\")"="UI: Update\nPaths: Prompt" ("State(s) in Front (\"\")"), "State(s) in (\"\")"=w350) -> ("States Out"=w349:string)  [unwired: 13 in]
      }
      frame "---------- Connection ----------" {
        # "Template Separator\n(You can make a copy of, or modify, this frame)"
        n142 = call <vilib>:"Add State(s) to Queue__jki_lib_state_machine.vi"("State(s) in (\"\")"=w354) -> ("States Out"=w353:string)  [unwired: 14 in]
      }
      frame "Connection: Close" {
        # "Template Separator\n(You can make a copy of, or modify, this frame)"
        n143 = Unbundle By Name(w358) -> ("Data.PG in"=w357:refnum<class "Data.PGSQL.lvclass">)
        n144 = call-dynamic "Close PG.vi"("error in (no error)"=w356, "Data.PG in"=w357) -> ("error out"=w355:errorcluster)  [unwired: 8 in, 1 out]
        n145 = call <vilib>:"Add State(s) to Queue__jki_lib_state_machine.vi"("State(s) in (\"\")"=w360) -> ("States Out"=w359:string)  [unwired: 14 in]
      }
      frame "Connection: Open" {
        # "Template Separator\n(You can make a copy of, or modify, this frame)"
        n146 = Unbundle By Name(w366) -> ("Data.PG in"=w364:refnum<class "Data.PGSQL.lvclass">)
        n147 = call "Set Connection Info.vi"("Data.PG in"=w364, "error in (no error)"=w361) -> ("Data.PG out"=w363:refnum<class "Data.PGSQL.lvclass">, "error out"=w362:errorcluster)  [unwired: 7 in]
        n148 = Bundle By Name(cluster=w366, "Data.PG in"=w363) -> (w365:T4)
        n149 = call <vilib>:"Add State(s) to Queue__jki_lib_state_machine.vi"("State(s) in (\"\")"=w368) -> ("States Out"=w367:string)  [unwired: 14 in]
      }
      frame "---------- Paths ----------" {
        # "Template Separator\n(You can make a copy of, or modify, this frame)"
        n150 = call <vilib>:"Add State(s) to Queue__jki_lib_state_machine.vi"("State(s) in (\"\")"=w372) -> ("States Out"=w371:string)  [unwired: 14 in]
      }
      frame "Paths: Get Table Path" {
        # "Template Separator\n(You can make a copy of, or modify, this frame)"
        n151 = Unbundle By Name(w379) -> ("Data.PG in"=w378:refnum<class "Data.PGSQL.lvclass">, "selected table"=w377:string)
        n152 = call "Get Table Path.vi"("error in (no error)"=w376, "Table"=w377, "Data.PG"=w378) -> ("error out"=w375:errorcluster, "Table Path"=w374:string)  [unwired: 6 in, 1 out]
        n153 = Bundle By Name(cluster=w379, "selected table path"=w374) -> (w373:T4)
        n154 = call <vilib>:"Add State(s) to Queue__jki_lib_state_machine.vi"("State(s) in (\"\")"=w381) -> ("States Out"=w380:string)  [unwired: 14 in]
      }
      frame "Paths: Get Column Path" {
        # "Template Separator\n(You can make a copy of, or modify, this frame)"
        n155 = Unbundle By Name(w393) -> ("Data.PG in"=w389:refnum<class "Data.PGSQL.lvclass">, "selected table path"=w382:string, "selected column"=w388:string, "selected table"=w392:string, "selected column"=w391:string)
        n156 = call "Get Column Path.vi"("error in (no error)"=w384, "Column"=w388, "Table path"=w382, "Data.PG in"=w389) -> ("error out"=w383:errorcluster, "Column Unit"=w386:string, "Column Path"=w387:string)  [unwired: 4 in, 1 out]
        n157 = call "Build Path.vi"("Table path"=w382, "Column path"=w387, "Table name"=w392, "Column name"=w391, "Column units"=w386) -> ("PG path"=→"path_to_selected_column":string)  [unwired: 10 in]
        n158 = Bundle By Name(cluster=w393, "selected column path"=w387, "selected column units"=w386) -> (w385:T4)
        n159 = call <vilib>:"Add State(s) to Queue__jki_lib_state_machine.vi"("State(s) in (\"\")"=w395) -> ("States Out"=w394:string)  [unwired: 14 in]
      }
      frame "Paths: Prompt" {
        # "Template Separator\n(You can make a copy of, or modify, this frame)"
        n160 = Unbundle By Name(w403) -> ("Current Index"=w398:i32, "Types (string)"=w400:string[], "Data"=w399:string[])
        n161 = Index Array(array=w400, index=w398) -> (element=w401:string)
        n162 = Index Array(array=w399, index=w398) -> (element=w397:string)
        n163 = Format Into String(format string="Element number --%d-- of data is of type --%s-- and has a value of --%s--.\nPlease double-click the column that stores this element", w398, w401, w397) -> (resulting string=w396:string)  [unwired: 2 in, 1 out]
        n164 = property on="Message" class="Str"("Text.Text"=w396) -> ()  [unwired: 2 in, 2 out]
        n165 = call <vilib>:"Add State(s) to Queue__jki_lib_state_machine.vi"("State(s) in (\"\")"=w406) -> ("States Out"=w405:string)  [unwired: 14 in]
      }
      frame "Paths: Add Path" {
        # "Template Separator\n(You can make a copy of, or modify, this frame)"
        n166 = Unbundle By Name(w419) -> ("Paths array"=w422:string[], "Current Index"=w417:i32, "Data"=w418:string[])
        n167 = Increment(x=w417) -> (x+1=w409:i32)
        n168 = Array Size(array=w418) -> (size(s)=w416:i32)
        n169 = Greater?(x=w409, y=4) -> (0:w413:bool)
        n170 = Equal?(x=w409, y=w416) -> (x = y?=w415:bool)
        n171 = case shown="True" w413 {
          tunnel: w409 -> [_ w429]
          tunnel: [0 w427] -> w410
          frame False {
          }
          frame True {
            n172 = Subtract(x=w429, y=4) -> (x-y=w427:i32)
          }
        }
        n173 = case shown="True" w415 {
          tunnel: w409 -> [w431 w434]
          tunnel: [w431 w432] -> w407
          tunnel: ["UI: Update Path Array\nPaths: Prompt" ("State(s) in Front (\"\")") "UI: Update Path Array\nUI: Finish\nMacro: Exit" ("State(s) in Front (\"\")")] -> w414
          frame False {
          }
          frame True {
            n174 = Decrement(x=w434) -> (x-1=w432:i32)
          }
        }
        n175 = property on="path_to_selected_column" class="Str"() -> ("Text.Text"=w421:string)  [unwired: 2 in, 2 out]
        n176 = Build Array(w410) -> (w411:i32[])
        n177 = property on="Paths" class="Arr (strict)"("Index Values"=w411) -> ()  [unwired: 2 in, 2 out]
        n178 = Insert Into Array(array=w422, new element=w421) -> (w420:string[])  [unwired: 1 in]
        n179 = Bundle By Name(cluster=w419, "Paths array"=w420, "Current Index"=w407) -> (w408:T4)
        n180 = call <vilib>:"Add State(s) to Queue__jki_lib_state_machine.vi"("State(s) in Front (\"\")"=w414, "State(s) in (\"\")"=w425) -> ("States Out"=w424:string)  [unwired: 13 in]
      }
      frame "Paths: Check If Okay" {
        # "Template Separator\n(You can make a copy of, or modify, this frame)"
        n181 = Unbundle By Name(w459) -> ("Paths array"=w458:string[], "Types (string)"=w452:string[], "Current Index"=w451:i32)
        n182 = property on="path_to_selected_column" class="Str"() -> ("Text.Text"=w442:string)  [unwired: 2 in, 2 out]
        n183 = call-poly <userlib>:"Search Array__ogtk.vi"("Array"=w458, "Element Data"=w442) -> ("Indices of Elements"=w457:i32[])  [unwired: 7 in]
        n184 = call "Parse Path Name.vi"("PG Path"=w442) -> ("Column path"=w441:string)  [unwired: 10 in, 4 out]
        n185 = Array Size(array=w457) -> (size(s)=w456:i32)
        n186 = String Subset(string=w441, offset (0)=0, length (rest)=1 ("length (rest)")) -> (substring=w439:string)
        n187 = Index Array(array=w452, index=w451) -> (element=w450:string)
        n188 = Equal To 0?(x=w456) -> (x = 0?=w455:bool)
        n189 = case shown="True" w455 {
          tunnel: [Errors--enum."5008: Cannot write two data points" ("Error code") Errors--enum."0: None" ("Error code")] -> w437
          frame False {
          }
          frame True {
          }
        }
        n190 = case shown="\"i\"" w439 {
          tunnel: w450 -> [_ w464 w468 w472 w476]
          tunnel: [Errors--enum."5005: Path Type Not Supported" ("Error code") w463 w467 w471 w475] -> w436
          frame "False", Default {
          }
          frame "v" {
            n191 = case shown="Default" w464 {
              tunnel: [Errors--enum."5050: Column can only hold string" ("Error code") Errors--enum."0: None" ("Error code")] -> w463
              frame Default {
              }
              frame "string" {
              }
            }
          }
          frame "b" {
            n192 = case shown="Default" w468 {
              tunnel: [Errors--enum."5051 Column can only hold bool" ("Error code") Errors--enum."0: None" ("Error code")] -> w467
              frame Default {
              }
              frame "boolean" {
              }
            }
          }
          frame "d" {
            n193 = case shown="Default" w472 {
              tunnel: [Errors--enum."5052: Column can only hold double" ("Error code") Errors--enum."0: None" ("Error code")] -> w471
              frame Default {
              }
              frame "double", "integer" {
              }
            }
          }
          frame "i" {
            n194 = case shown="Default" w476 {
              tunnel: [Errors--enum."5053: Column can only hold int" ("Error code") Errors--enum."0: None" ("Error code")] -> w475
              frame Default {
              }
              frame "integer" {
              }
            }
          }
        }
        n195 = call "Error Handler.vi"("Error code"=w437) -> ("error out"=w438:errorcluster)
        n196 = call "Error Handler.vi"("Error code"=w436) -> ("error out"=w435:errorcluster)
        n197 = Merge Errors(w438, w435, w440) -> (w449:errorcluster)
        n198 = call <vilib>:"Simple Error Handler.vi"("error in (no error)"=w449) -> ("error?"=w446:bool, "error out"=w444:errorcluster)  [unwired: 4 in, 3 out]
        n199 = Select(t="", s=w446, f="Paths: Add Path") -> (s? t:f=w445:string)
        n200 = call <vilib>:"Clear Errors.vi"("error in (no error)"=w444) -> ("error out"=w443:errorcluster)  [unwired: 6 in]
        n201 = call <vilib>:"Add State(s) to Queue__jki_lib_state_machine.vi"("State(s) in Front (\"\")"=w445, "State(s) in (\"\")"=w461) -> ("States Out"=w460:string)  [unwired: 13 in]
      }
    }
  }
